vi "Find.vi"(8 "Error In":errorcluster, 10 "Key":string, 11 "Renderer In":refnum<class "Renderer.lvclass">) -> (0 "Error Out":errorcluster, 1 "Found?":bool, 2 "Datum":refnum<class "Datum.lvclass">, 3 "Renderer Out":refnum<class "Renderer.lvclass">)   [LabVIEW 2018, in "Toolkit.lvlib" / "Renderer.lvclass"]
doc: "Finds a value associated with the key within the context."
uses:
  Renderer.lvclass
  Data/Datum/Datum.lvclass
  Renderer.lvclass/Renderer.ctl
  Data/Null/Null.lvclass
  D:/Users/cfield/Code/Field R&D Services/Labstache/src/Toolkit/Data/Datum/Datum.lvclass
  Data/Map/Map.lvclass
  Data/Pair/Pair.lvclass
  Data/Pair/Pair.lvclass/Pair.ctl
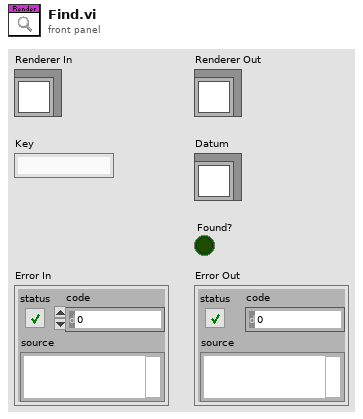
[diagram p1: front panel]
types:
  T1 = typedef "Toolkit.lvlib/Data.lvlib/Types.ctl" = enum16{"Array", "Boolean", "Function", "Map", "Null", "Pair", "Path", "String", "Unknown"}
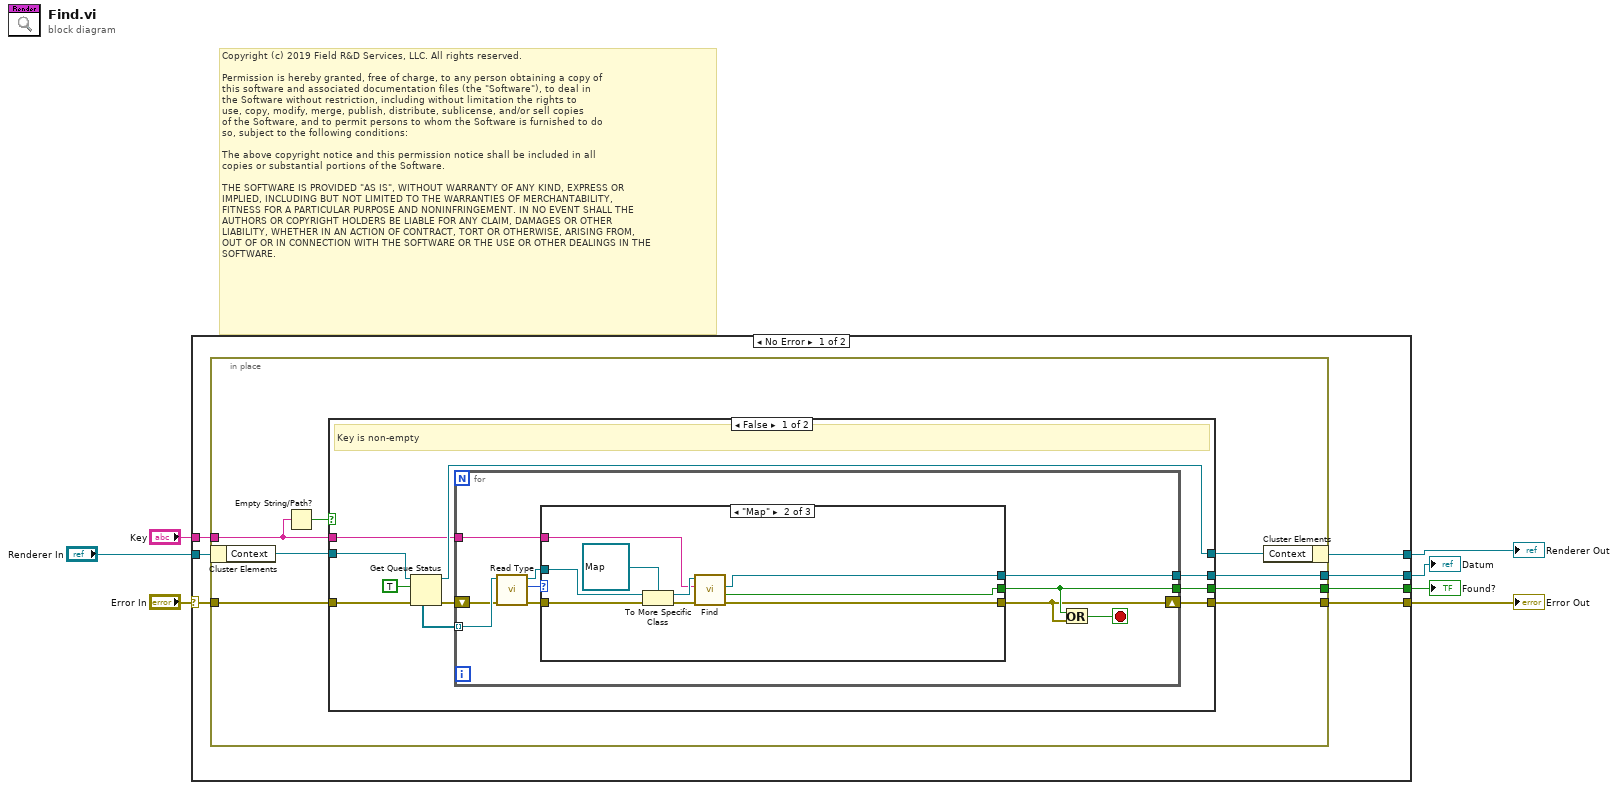
[diagram p0: block diagram]
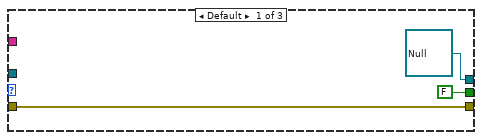
[diagram p2: hidden frame]
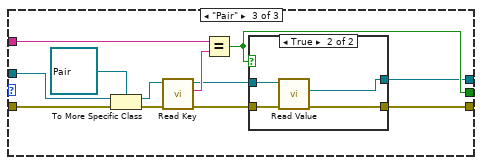
[diagram p3: hidden frame]
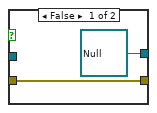
[diagram p4: hidden frame]
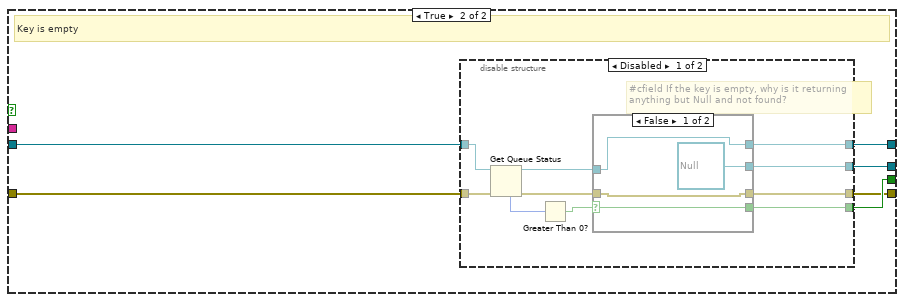
[diagram p5: hidden frame]
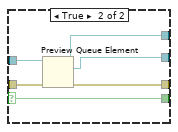
[diagram p6: hidden frame]
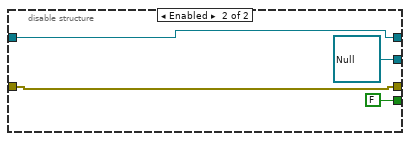
[diagram p7: hidden frame]
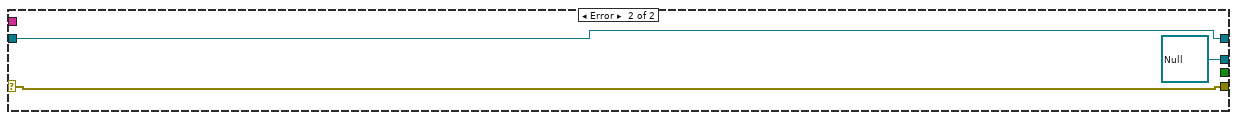
[diagram p8: hidden frame]
diagram:
  # "Copyright (c) 2019 Field R&D Services, LLC. All rights reserved.\n\nPermission is hereby granted, free of charge, to any person obtaining a copy of\nthis software and associated documentation files (the \"Software\"), to deal in\nthe Software without restriction, including without limitation the rights to\nuse, copy, modify, merge, publish, distribute, sublicense, and/or sell copies\nof the Software, and to permit persons to whom the Software is furnished to do\nso, subject to the following conditions:\n\nThe above copyright notice and this permission notice shall be included in all\ncopies or substantial portions of the Software.\n\nTHE SOFTWARE IS PROVIDED \"AS IS\", WITHOUT WARRANTY OF ANY KIND, EXPRESS OR\nIMPLIED, INCLUDING BUT NOT LIMITED TO THE WARRANTIES OF MERCHANTABILITY,\nFITNESS FOR A PARTICULAR PURPOSE AND NONINFRINGEMENT. IN NO EVENT SHALL THE\nAUTHORS OR COPYRIGHT HOLDERS BE LIABLE FOR ANY CLAIM, DAMAGES OR OTHER\nLIABILITY, WHETHER IN AN ACTION OF CONTRACT, TORT OR OTHERWISE, ARISING FROM,\nOUT OF OR IN CONNECTION WITH THE SOFTWARE OR THE USE OR OTHER DEALINGS IN THE\nSOFTWARE."
  n1 = case shown="No Error" "Error In" {
    selector: "Error In" -> [w11 w104]
    tunnel: [w14 refnum<class "Null.lvclass"> refnum ("Toolkit.lvlib:Data.lvlib:Null.lvclass")] -> w7
    tunnel: [w13 w104] -> w6
    tunnel: [w12 _] -> w5
    tunnel: "Renderer In" -> [w10 w105]
    tunnel: [w9 w105] -> w1
    tunnel: "Key" -> [w8 _]
    frame No Error {
      n2 = in-place {
        in-place-border: [w22] -> w14
        in-place-border: [w21] -> w13
        in-place-border: [w20] -> w12
        in-place-border: w11 -> [w19]
        in-place-border: w8 -> [w16]
        n3 = in-place-cluster #1(w10) -> ("Context"=w18:refnum<queue>)
        n4 = Empty String/Path?(string/path=w16) -> (empty?=w15:bool)
        n5 = case shown="False" w15 {
          tunnel: [w32 w77] -> w22
          tunnel: [w31 w73] -> w21
          tunnel: [w27 w74] -> w20
          tunnel: w19 -> [w26 w75]
          tunnel: w18 -> [w25 w76]
          tunnel: [w24 w78] -> w17
          tunnel: w16 -> [w23 _]
          frame False {
            # "Key is non-empty"
            n6 = Get Queue Status(queue=w25, return elements? (F)=TRUE, error in (no error)=w26) -> (queue out=w24:refnum<queue>, error out=w30:errorcluster, elements=w29:refnum<class "Datum.lvclass">[])  [unwired: 5 out]
            n7 = for {
              tunnel: w29 -> [w40] mode=indexing
              tunnel: w23 -> [w42]
              tunnel: [w41] -> w32
              tunnel: [w35] -> w27
              shift-right: [w34] -> w31
              shift-left: w30 -> [w38]
              stop <- w33 stop-if-true
              n8 = call-dynamic "Read Type.vi"("Error In"=w38, "Datum In"=w40) -> ("Error Out"=w37:errorcluster, "Type"=w36:T1, "Datum Out"=w39:refnum<class "Datum.lvclass">)  [unwired: 7 in]
              n9 = case shown="\"Map\"" w36 {
                tunnel: w37 -> [w44 w54 w66]
                tunnel: w39 -> [_ w53 w65]
                tunnel: w42 -> [_ w49 w60]
                tunnel: [w44 w48 w57] -> w34
                tunnel: [FALSE ("Found?") w46 w59] -> w35
                tunnel: [refnum<class "Null.lvclass"> refnum ("Toolkit.lvlib:Data.lvlib:Null.lvclass") w47 w55] -> w41
                frame Default {
                }
                frame "Map" {
                  n10 = To More Specific Class(target class=refnum<class "Map.lvclass"> refnum ("Toolkit.lvlib:Data.lvlib:Map.lvclass"), reference=w53, error in=w54) -> (specific class reference=w50:refnum<class "Map.lvclass">, error out=w51:errorcluster)
                  n11 = call "Find.vi"("Error In"=w51, "Key"=w49, "Map In"=w50) -> ("Error Out"=w48:errorcluster, "Found?"=w46:bool, "Value"=w47:refnum<class "Datum.lvclass">)  [unwired: 5 in, 1 out]
                }
                frame "Pair" {
                  n12 = To More Specific Class(target class=refnum<class "Pair.lvclass"> refnum ("Toolkit.lvlib:Data.lvlib:Pair.lvclass"), reference=w65, error in=w66) -> (specific class reference=w63:refnum<class "Pair.lvclass">, error out=w62:errorcluster)
                  n13 = call "Read Key.vi"("Error In"=w62, "Pair In"=w63) -> ("Error Out"=w58:errorcluster, "Key"=w61:string, "Pair Out"=w56:refnum<class "Pair.lvclass">)  [unwired: 7 in]
                  n14 = Equal?(x=w60, y=w61) -> (x = y?=w59:bool)
                  n15 = case shown="True" w59 {
                    tunnel: w58 -> [w68 w72]
                    tunnel: [w68 w71] -> w57
                    tunnel: w56 -> [_ w70]
                    tunnel: [refnum<class "Null.lvclass"> refnum ("Toolkit.lvlib:Data.lvlib:Null.lvclass") w69] -> w55
                    frame False {
                    }
                    frame True {
                      n16 = call "Read Value.vi"("Error In"=w72, "Pair In"=w70) -> ("Error Out"=w71:errorcluster, "Value"=w69:refnum<class "Datum.lvclass">)  [unwired: 7 in, 1 out]
                    }
                  }
                }
              }
              n17 = Or(x=w35, y=w34) -> (x .or. y?=w33:bool)
            }
          }
          frame True {
            # "Key is empty"
            n18 = disable-structure "Diagram Disable Structure" shown="Disabled" {
              disable-tunnel: [w88 w102] -> w78
              disable-tunnel: [w87 refnum<class "Null.lvclass"> refnum ("Toolkit.lvlib:Data.lvlib:Null.lvclass")] -> w77
              disable-tunnel: w76 -> [w86 w102]
              disable-tunnel: w75 -> [w83 w101]
              disable-tunnel: [w80 FALSE] -> w74
              disable-tunnel: [w79 w101] -> w73
              frame Disabled {
                # "#cfield If the key is empty, why is it returning anything but Null and not found?"
                n19 = Get Queue Status(queue=w86, error in (no error)=w83) -> (queue out=w85:refnum<queue>, error out=w84:errorcluster, # elements in queue=w82:i32)  [unwired: 1 in, 5 out]
                n20 = Greater Than 0?(x=w82) -> (x > 0?=w81:bool)
                n21 = case shown="False" w81 {
                  selector: w81 -> [w91 w93]
                  tunnel: [w92 w98] -> w88
                  tunnel: [refnum<class "Null.lvclass"> refnum ("Toolkit.lvlib:Data.lvlib:Null.lvclass") w97] -> w87
                  tunnel: w85 -> [w92 w96]
                  tunnel: w84 -> [w90 w95]
                  tunnel: [w91 w93] -> w80
                  tunnel: [w90 w94] -> w79
                  frame False {
                  }
                  frame True {
                    n22 = Preview Queue Element(queue=w96, error in (no error)=w95) -> (queue out=w98:refnum<queue>, element=w97:refnum<class "Datum.lvclass">, error out=w94:errorcluster)  [unwired: 1 in, 1 out]
                  }
                }
              }
              frame Enabled {
              }
            }
          }
        }
        n23 = in-place-cluster #1("Context"=w17) -> (w9:refnum<class "Renderer.lvclass">)
      }
    }
    frame Error {
    }
  }
  "Datum" <- w7
  "Error Out" <- w6
  "Found?" <- w5
  "Renderer Out" <- w1
